vi "Sequencer.min.vi"() -> ()   [LabVIEW 2014]
uses:
  <vilib>/Analysis/NI_AALPro.lvlib
panel:
  in  "Trigger":bool
  out "Counts":u32[](array[numeric])
  out "PMT4":u32[](array[numeric])
  out "PMT3":u32[](array[numeric])
  out "PMT2":u32[](array[numeric])
  out "PMT1":u32[](array[numeric])
  in  "Threshold":dbl=1.0
  out "CompiledSequence":string="#DopplerCooling\r\n0.9 10100000 00000000 00000000\r\n\r\n#Pump\r\n0.3 01000000 00000000 00000000\r\n\r\n#Pulsed\r\n0.2 00100000 00000000 00000000\r\n0.4 00000100 00000000 00000000\r\n0.2 00000000 10000000 00000000\r\n0.2 01000000 00000000 01000000\n"
  out "ChapterNames":string[](array[string])
  out "ChapterPositions":u32[](array[numeric])
  in  "Scan":enum32{"Time"}(tab)
  out "Now (us)":dbl=1.0 format="%.2f"
  in  "Step (us)":dbl=1.0 format="%.2f"
  in  "End (us)":dbl=1.0 format="%.2f"
  in  "Start (us)":dbl=1.0 format="%.2f"
  in  "Time Scan":bool
  in  "Chapter":u16(ring) items=["Zero", "Cooling[0]", "Cooling[1]", "Cooling[2]", "Zero"]
  in  "Once":bool=TRUE
  in  "Sequencer Port":refnum<visa-resource-name>="COM5"
  in  "Send":bool
  out "Durations Backup":dbl[](array[numeric])
  out "Durations":dbl[](array[numeric])
  in  "Period (ns)":dbl=5.0
  out "States":string[](array[string])
  in  "Sequencer":bool
  in  "Edit":enum32{"Sequence"}(tab)
  in  "Sequence":string
  in  "Save":bool
  in  "Chapter (us)":string
  in  "Sequence File":path=path "E:/Data/Sequence/Cooling.seq"
  in  "Repeats":u32=100
  in  "Compile":bool
  in  "Data":bool
  out "Clock":string
  in  "Detect":enum32{"PMT", "TTL"}(tab)
  in  "4":bool
  in  "3":bool
  in  "2":bool
  in  "1":bool=TRUE
  in  "Save":bool
  in  "Count or State":i16(ring) items=["Count", "State"]
  in  "Fit":bool
  out "Peak":u32
  out "?":cluster{dbl[], "Axis":dbl[]}(graph)
  out "?":cluster{"Axis":dbl[], "Histogram":i32[]}(graph)
  in  "Data Chapter":i16(ring) items=["All", "Cooling[2]"]
  out "Average Counts or States":dbl(graph)
  out "Average of Scans":dbl[](graph)
  out "data file":string
  out "History Data":dbl[](array[numeric])
  in  "Sweep":bool
  in  "Clear":bool
  out "Digital Waveform Graph":digitaldata(graph)
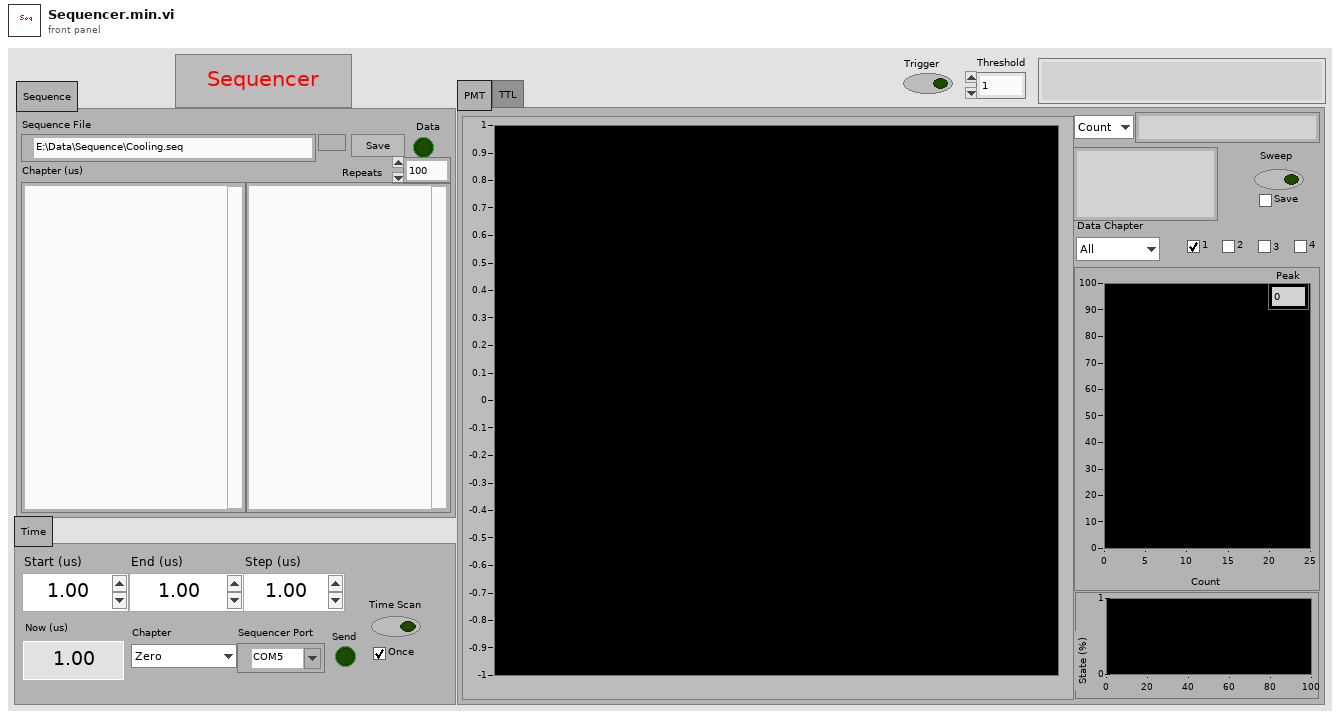
[diagram p1: front panel]
types:
  T1 = cluster{"lower":dbl, "upper":dbl, "inclusion":enum32{"lower", "upper", "both", "neither"}}[]
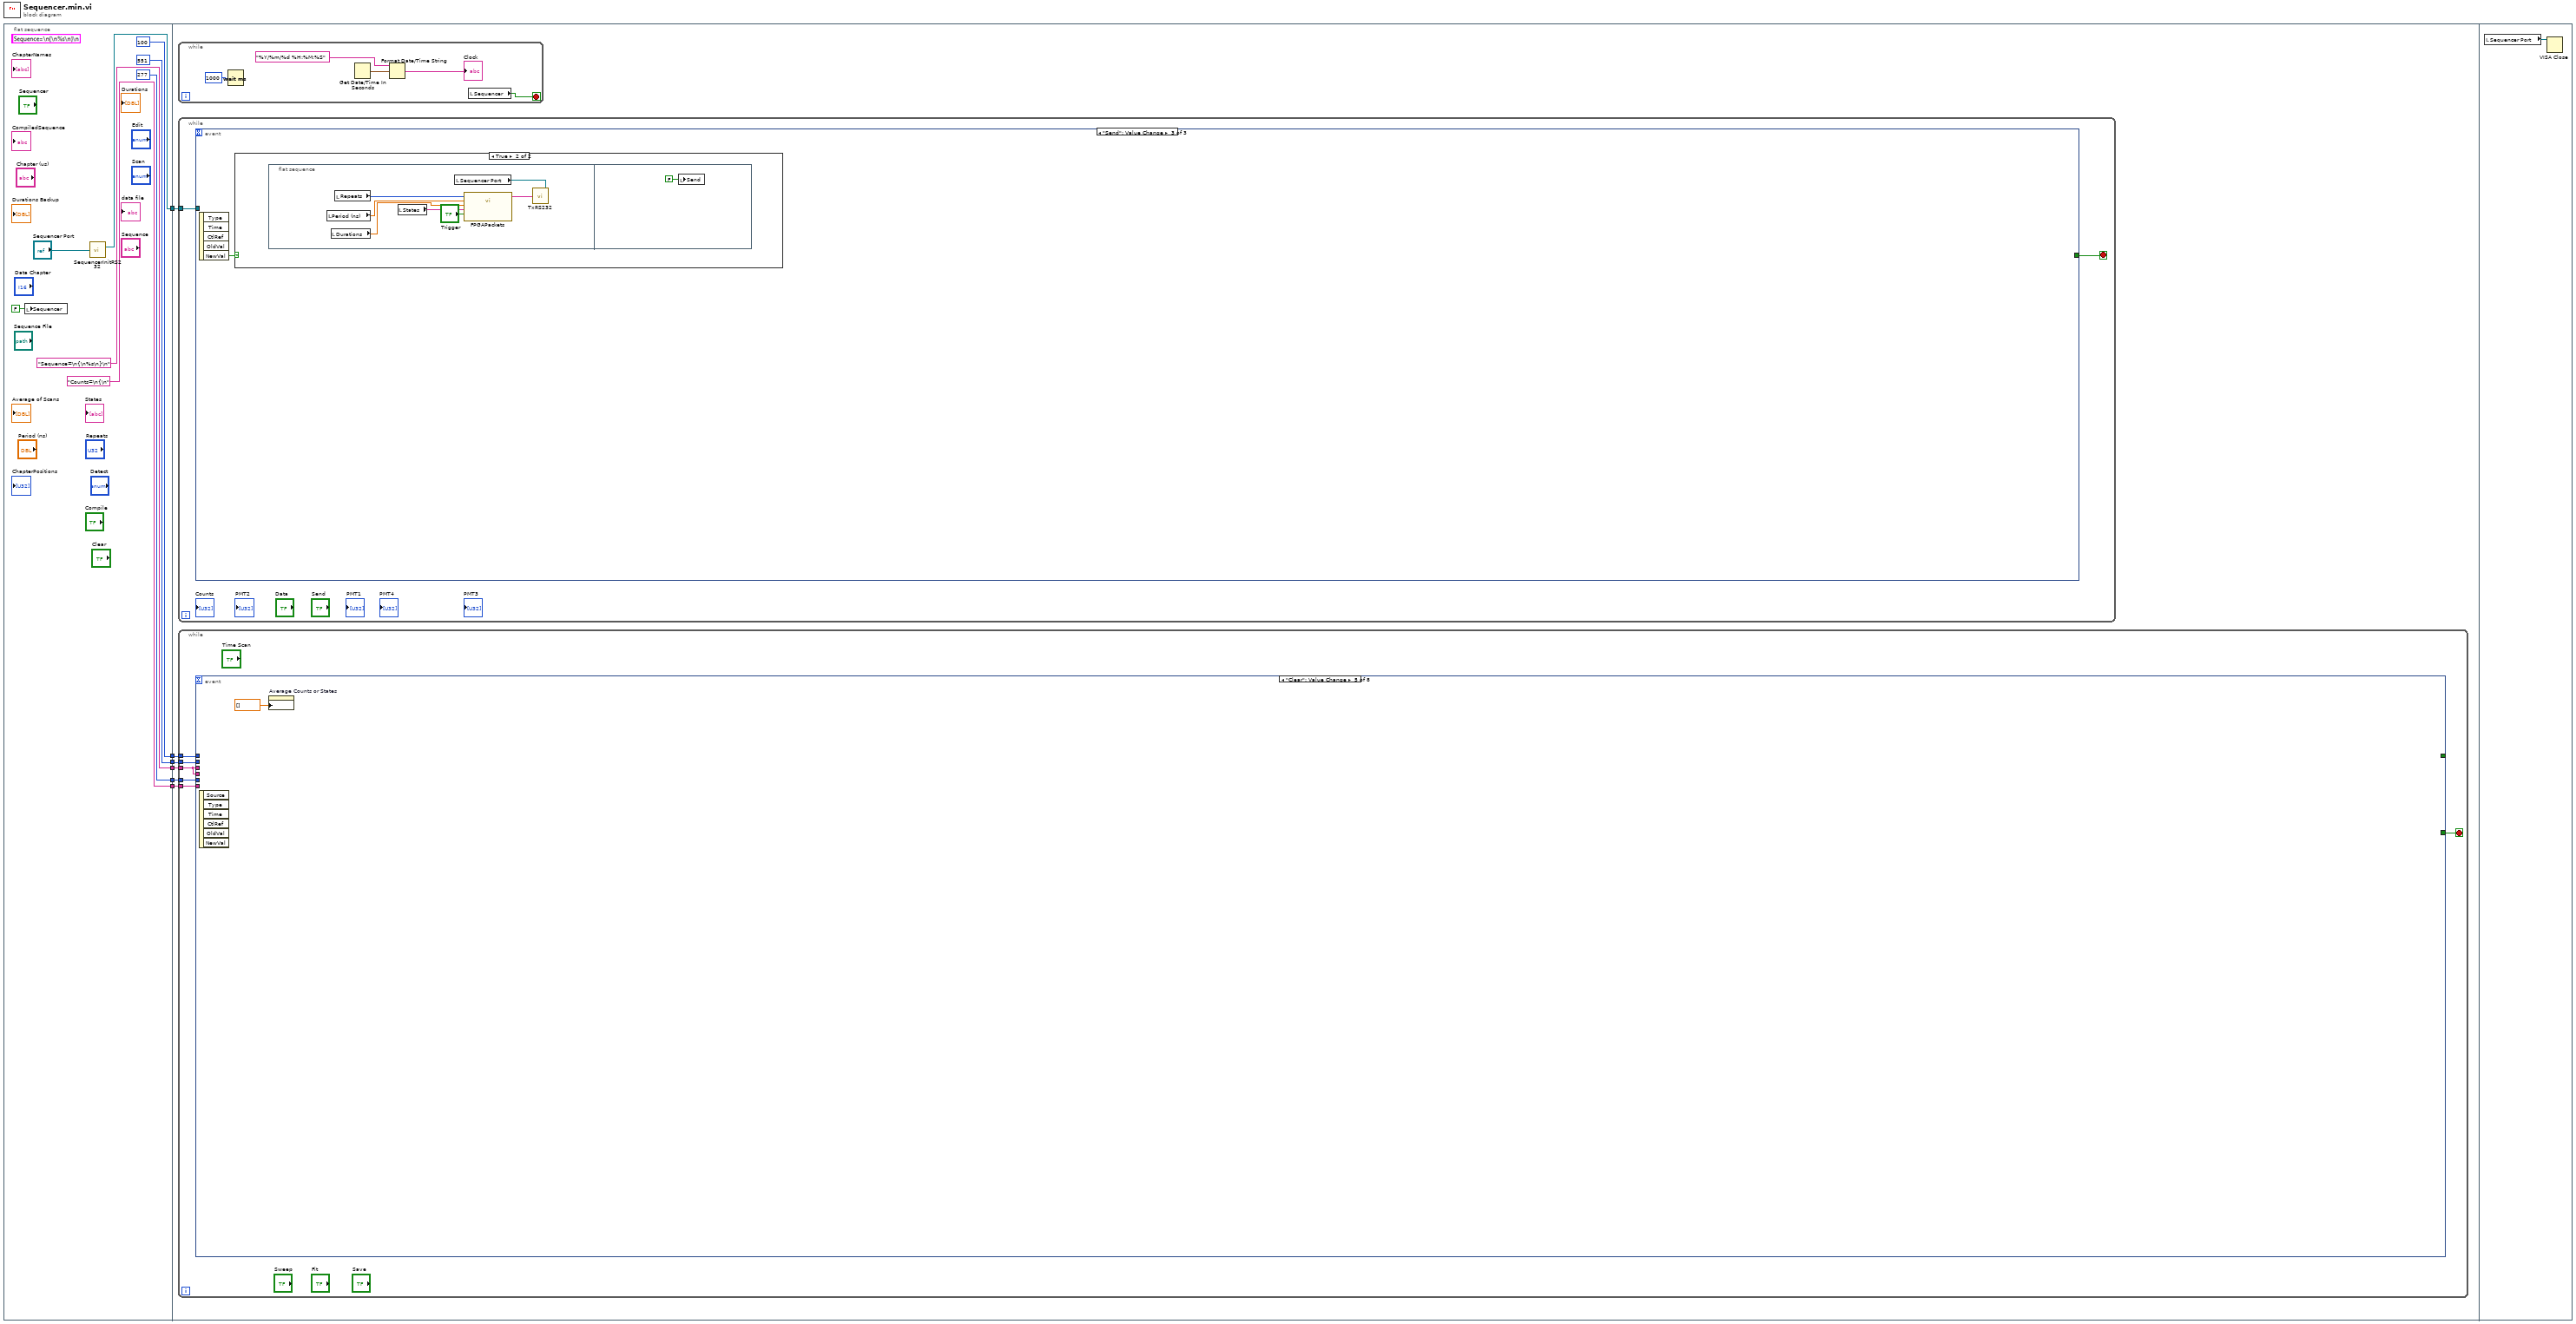
[diagram p0: block diagram]
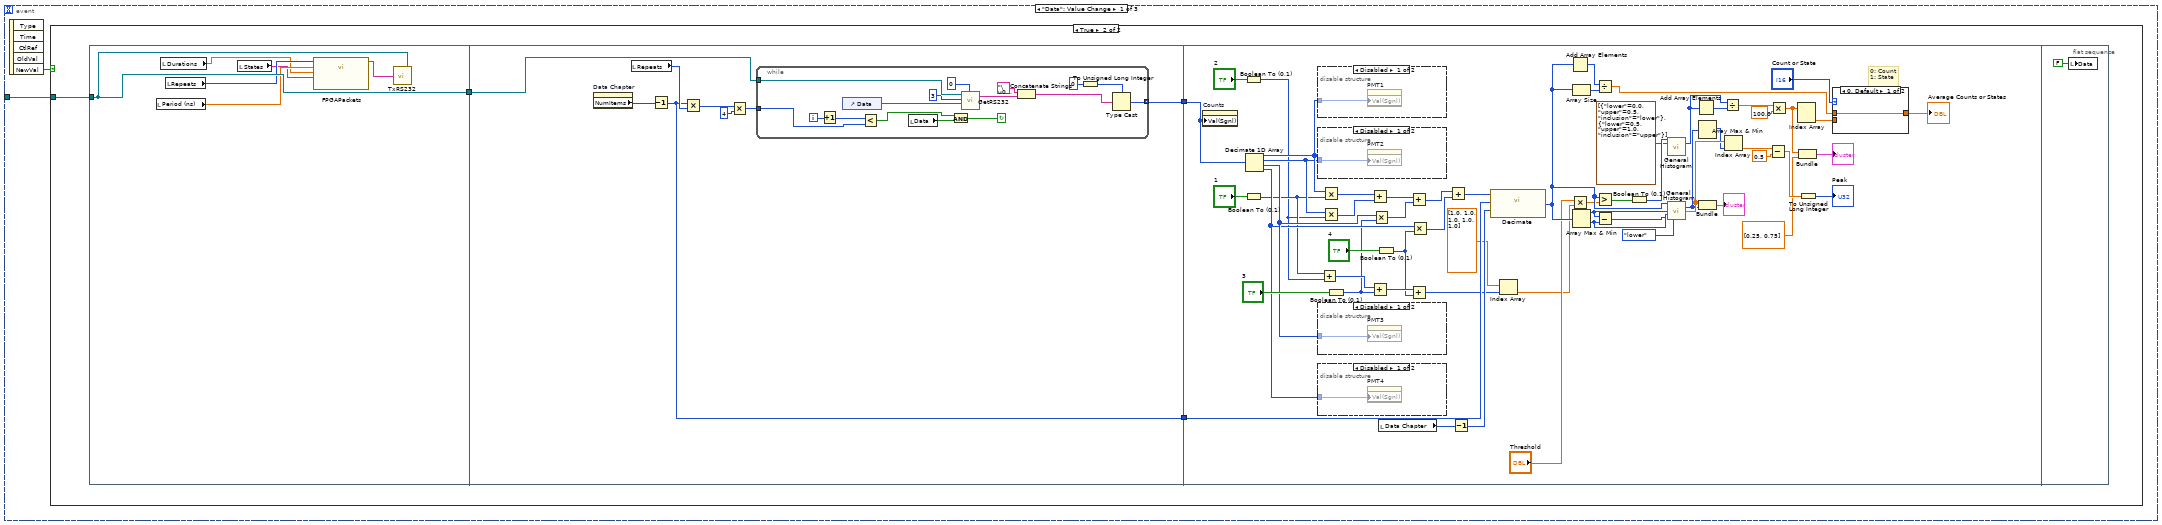
[diagram p2: hidden frame]
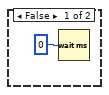
[diagram p3: hidden frame]
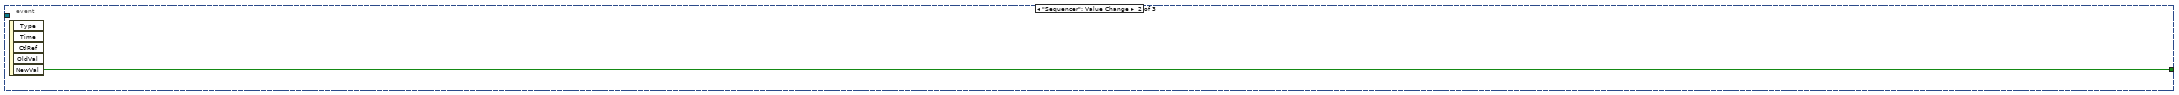
[diagram p9: hidden frame]
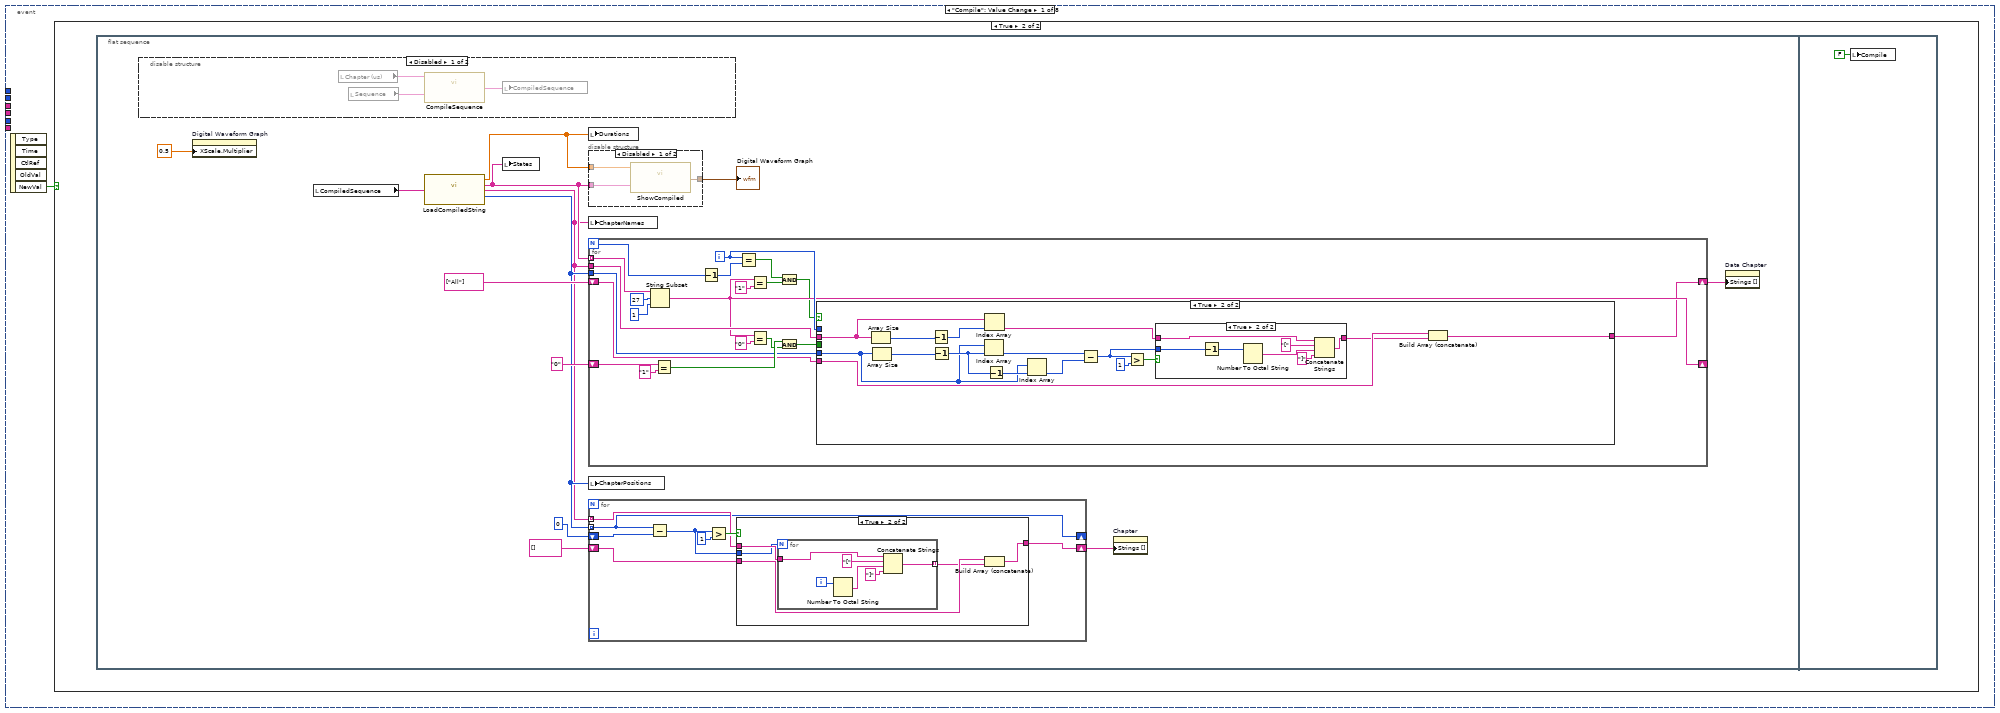
[diagram p11: hidden frame]
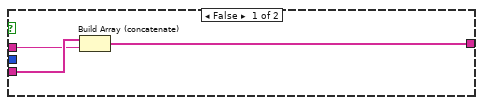
[diagram p15: hidden frame]
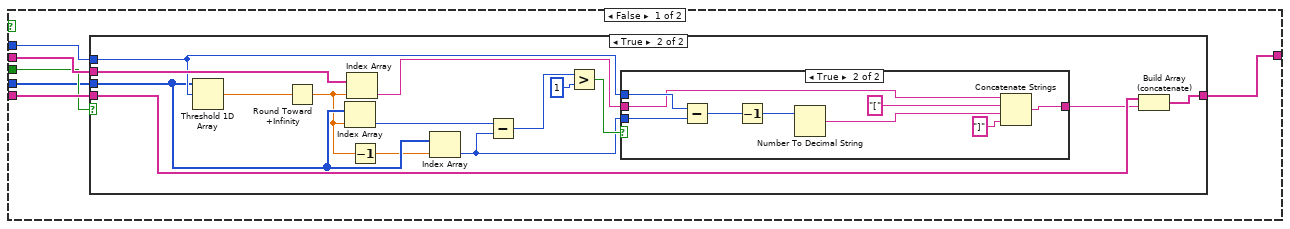
[diagram p16: hidden frame]
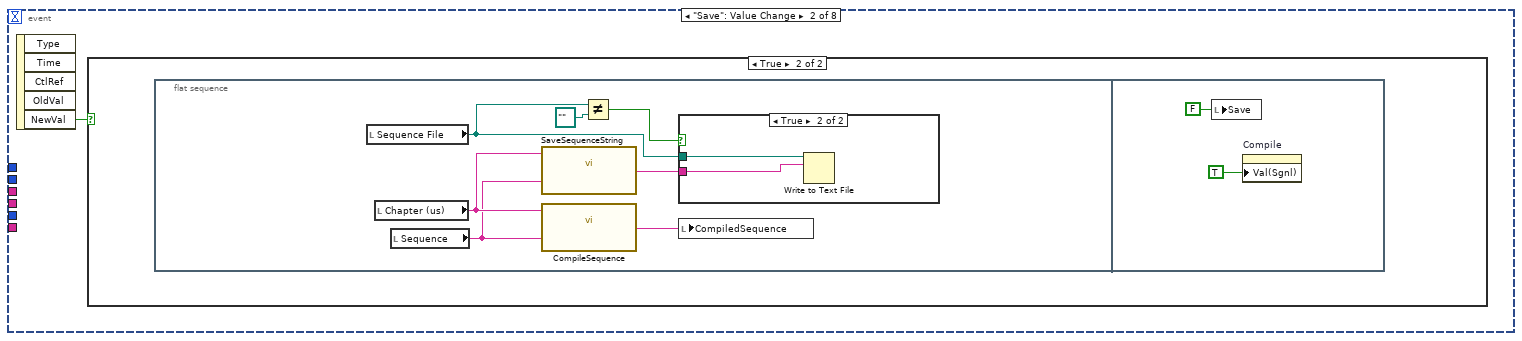
[diagram p20: hidden frame]
diagram:
  n1 = flat-sequence {
    tunnel: [w7] -> w6
    tunnel: [u32 277 ("XControl:Container Bounds:Height")] -> w5
    tunnel: [u32 551 ("Plot Area:Size:Height")] -> w4
    tunnel: [100 ("y")] -> w3
    tunnel: ["Sequence=\n{\n%s\n}\n" ("format string")] -> w2
    tunnel: ["Counts=\n{\n" ("text")] -> w1
    tunnel: w6 -> [w20]
    tunnel: w5 -> [w19]
    tunnel: w4 -> [w18]
    tunnel: w3 -> [w17]
    tunnel: w2 -> [w16]
    tunnel: w1 -> [w15]
    frame #0 {
      n2 = local write "Sequencer"(FALSE ("Sequencer")) -> ()
      n3 = call "SequencerInitRS232.vi"("VISA resource name"="Sequencer Port") -> ("reference out"=w7:refnum<visa-resource-name>)  [unwired: 1 out]
    }
    frame #1 {
      n4 = while {
        stop <- w21 stop-if-true
        n5 = Wait (ms)(milliseconds to wait=u32 1000) -> ()  [unwired: 1 out]
        n6 = Get Date/Time In Seconds() -> (seconds since 1Jan1904=w25:timestamp)
        n7 = Format Date/Time String(time format string (%c)="%Y/%m/%d %H:%M:%S", seconds (now)=w25) -> (date/time string=→"Clock":string)  [unwired: 1 in]
        n8 = local read "Sequencer"() -> (w21:bool)
      }
      n9 = while {
        tunnel: w20 -> [w27]
        stop <- w26 stop-if-true
        n10 = event shown="[2] \"Send\": Value Change" {
          selector: _ -> [_ _ _]
          dyn-events: _ -> [_ _ _]
          timeout: _ -> [_ _ _]
          tunnel: w27 -> [w29 _ _]
          tunnel: [_ w131 _] -> w26
          event "Data": Value Change {
            n11 = event-data() -> ("NewVal"=w28:bool)  [unwired: 1 in, 4 out]
            n12 = case shown="True" w28 {
              tunnel: w29 -> [_ w34]
              frame False {
                n13 = Wait (ms)(milliseconds to wait=u32 0) -> ()  [unwired: 1 out]
              }
              frame True {
                n14 = flat-sequence {
                  tunnel: w34 -> [w39]
                  tunnel: [w39] -> w31
                  tunnel: [w46] -> w33
                  tunnel: [w44] -> w32
                  tunnel: w31 -> [w48]
                  tunnel: w33 -> [w91]
                  tunnel: w32 -> [w97]
                  frame #0 {
                    n15 = local read "Period (ns)"() -> (w37:dbl)
                    n16 = local read "Durations"() -> (w36:dbl[])
                    n17 = local read "Repeats"() -> (w38:u32)
                    n18 = local read "States"() -> (w35:string[])
                    n19 = call "FPGAPackets.vi"("Repeats"=w38, "Period (ns)"=w37, "Durations"=w36, "States"=w35) -> ("Packets"=w40:string)  [unwired: 1 in, 1 out]
                    n20 = call "TxRS232.vi"("VISA resource name"=w39, "Data"=w40) -> ()
                  }
                  frame #1 {
                    n21 = property on="Data Chapter" class="Ring (strict)"() -> ("NumItems"=w47:u32)  [unwired: 2 in, 2 out]
                    n22 = local read "Repeats"() -> (w45:u32)
                    n23 = Decrement(x=w47) -> (x-1=w44:u32)
                    n24 = Multiply(x=w44, y=w45) -> (x*y=w43:u32)
                    n25 = Multiply(x=w43, y=u32 4) -> (x*y=w42:u32)
                    n26 = while {
                      tunnel: w48 -> [w56]
                      tunnel: [w57] -> w46 mode=indexing
                      tunnel: w42 -> [w52]
                      i -> [w51]
                      stop <- w60 continue-if-true
                      n27 = Increment(x=w51) -> (x+1=w50:i32)
                      n28 = control-ref of="Data"() -> (w53:refnum<vi>)
                      n29 = Less?(x=w50, y=w52) -> (x < y?=w59:bool)
                      n30 = local read "Data"() -> (w61:bool)
                      n31 = And(x=w59, y=w61) -> (x .and. y?=w60:bool)
                      n32 = call "GetRS232.vi"("VISA resource name"=w56, "Bytes To Read"=3, "Control"=w53, "Limit"=0) -> ("Data"=w54:string)  [unwired: 1 in, 1 out]
                      n33 = Concatenate Strings("\u0000" ("string"), w54) -> (w58:string)
                      n34 = To Unsigned Long Integer(number=u32 0) -> (unsigned 32bit integer=w64:u32)
                      n35 = Type Cast(type=w64, x=w58) -> (*(type *) &x=w57:u32)
                    }
                  }
                  frame #2 {
                    # "0: Count\n1: State"
                    n36 = property on="Counts" class="Arr (strict)"("Val(Sgnl)"=w91) -> ()  [unwired: 2 in, 2 out]
                    n37 = Boolean To (0,1)(Boolean="2") -> (0, 1=w74:i16)
                    n38 = Boolean To (0,1)(Boolean="1") -> (0, 1=w75:i16)
                    n39 = Decimate 1D Array(w91) -> (w90:u32[], w87:u32[], w83:u32[], w80:u32[])
                    n40 = disable-structure shown="Disabled" {
                      disable-tunnel: w90 -> [w127 _]
                      frame Disabled {
                        n41 = property on="PMT1" class="Arr (strict)"("Val(Sgnl)"=w127) -> ()  [unwired: 2 in, 2 out]
                      }
                      frame Enabled {
                      }
                    }
                    n42 = disable-structure shown="Disabled" {
                      disable-tunnel: w87 -> [w126 _]
                      frame Disabled {
                        n43 = property on="PMT2" class="Arr (strict)"("Val(Sgnl)"=w126) -> ()  [unwired: 2 in, 2 out]
                      }
                      frame Enabled {
                      }
                    }
                    n44 = disable-structure shown="Disabled" {
                      disable-tunnel: w83 -> [w125 _]
                      frame Disabled {
                        n45 = property on="PMT3" class="Arr (strict)"("Val(Sgnl)"=w125) -> ()  [unwired: 2 in, 2 out]
                      }
                      frame Enabled {
                      }
                    }
                    n46 = disable-structure shown="Disabled" {
                      disable-tunnel: w80 -> [w124 _]
                      frame Disabled {
                        n47 = property on="PMT4" class="Arr (strict)"("Val(Sgnl)"=w124) -> ()  [unwired: 2 in, 2 out]
                      }
                      frame Enabled {
                      }
                    }
                    n48 = Add(x=w75, y=w74) -> (x+y=w73:i16)
                    n49 = Multiply(x=w90, y=w75) -> (x*y=w76:u32[])
                    n50 = Multiply(x=w87, y=w74) -> (x*y=w86:u32[])
                    n51 = Boolean To (0,1)(Boolean="3") -> (0, 1=w72:i16)
                    n52 = Add(x=w76, y=w86) -> (x+y=w81:u32[])
                    n53 = Add(x=w73, y=w72) -> (x+y=w71:i16)
                    n54 = Multiply(x=w83, y=w72) -> (x*y=w82:u32[])
                    n55 = Boolean To (0,1)(Boolean="4") -> (0, 1=w70:i16)
                    n56 = local read "Data Chapter"() -> (w95:i16)
                    n57 = Add(x=w81, y=w82) -> (x+y=w78:u32[])
                    n58 = Add(x=w71, y=w70) -> (x+y=w65:i16)
                    n59 = Multiply(x=w80, y=w70) -> (x*y=w79:u32[])
                    n60 = Add(x=w78, y=w79) -> (x+y=w77:u32[])
                    n61 = Decrement(x=w95) -> (x-1=w94:i16)
                    n62 = call "Decimate.vi"("i"=w94, "n"=w97, "Input Array"=w77) -> ("Decimated Array"=w119:u32[])
                    n63 = Index Array(array=dbl[] [1.0, 1.0, 1.0, 1.0, 1.0], index=w65) -> (element=w67:dbl)
                    n64 = Add Array Elements(numeric array=w119) -> (sum=w118:u32)
                    n65 = Multiply(x="Threshold", y=w67) -> (x*y=w66:dbl)
                    n66 = Array Size(array=w119) -> (size(s)=w117:i32)
                    n67 = Array Max & Min(array=w119) -> (max value=w98:u32, min value=w108:u32)  [unwired: 2 out]
                    n68 = Divide(x=w118, y=w117) -> (x/y=w121:dbl)
                    n69 = Greater?(x=w119, y=w66) -> (0:w104:bool[])
                    n70 = Subtract(x=w98, y=w108) -> (x-y=w107:u32)
                    n71 = Boolean To (0,1)(Boolean=w104) -> (0, 1=w103:i16[])
                    n72 = call <vilib>:"General Histogram.vi"("X"=w103, "Bins"=T1 [{"lower"=0.0, "upper"=0.5, "inclusion"=enum."lower"}, {"lower"=0.5, "upper"=1.0, "inclusion"=enum."upper"}]) -> ("Histogram"=w101:i32[])  [unwired: 9 in, 4 out]
                    n73 = call <vilib>:"General Histogram.vi"("X"=w119, "max"=w98, "min"=w108, "# bins"=w107, "inclusion"=enum32{"lower", "upper"}."lower") -> ("Histogram"=w109:i32[], "Axis"=w111:dbl[])  [unwired: 6 in, 3 out]
                    n74 = Add Array Elements(numeric array=w101) -> (sum=w102:i32)
                    n75 = Array Max & Min(array=w109) -> (max index (indices)=w110:i32)  [unwired: 3 out]
                    n76 = Bundle("Axis"=w111, "Histogram"=w109) -> (→"?":cluster{"Axis":dbl[], "Histogram":i32[]})  [unwired: 1 in]
                    n77 = Divide(x=w101, y=w102) -> (x/y=w99:dbl[])
                    n78 = Index Array(array=w111, index=w110) -> (element=w115:dbl)
                    n79 = Subtract(x=w115, y=0.5) -> (x-y=w114:dbl)
                    n80 = Multiply(x=w99, y=100.0) -> (x*y=w120:dbl[])
                    n81 = Index Array(array=w120) -> (element #2=w122:dbl)  [unwired: 2 in, 1 out]
                    n82 = Bundle(w120, "Axis"=dbl[] [0.25, 0.75]) -> (→"?":cluster{dbl[], "Axis":dbl[]})  [unwired: 1 in]
                    n83 = To Unsigned Long Integer(number=w114) -> (unsigned 32bit integer=→"Peak":u32)
                    n84 = case shown="0, Default" "Count or State" {
                      tunnel: w121 -> [w128 _]
                      tunnel: [w128 w129] -> w123
                      tunnel: w122 -> [_ w129]
                      frame 0, Default {
                      }
                      frame 1 {
                      }
                    }
                    "Average Counts or States" <- w123
                  }
                  frame #3 {
                    n85 = local write "Data"(FALSE ("Acquisition")) -> ()
                  }
                }
              }
            }
          }
          event "Sequencer": Value Change {
            n86 = event-data() -> ("NewVal"=w131:bool)  [unwired: 1 in, 4 out]
          }
          event "Send": Value Change {
            n87 = event-data() -> ("NewVal"=w132:bool)  [unwired: 1 in, 4 out]
            n88 = case shown="True" w132 {
              frame False {
              }
              frame True {
                n89 = flat-sequence {
                  frame #0 {
                    n90 = local read "Period (ns)"() -> (w137:dbl)
                    n91 = local read "Durations"() -> (w135:dbl[])
                    n92 = local read "Repeats"() -> (w136:u32)
                    n93 = local read "States"() -> (w138:string[])
                    n94 = local read "Sequencer Port"() -> (w139:refnum<visa-resource-name>)
                    n95 = call "FPGAPackets.vi"("Repeats"=w136, "Period (ns)"=w137, "Durations"=w135, "States"=w138, "Trigger"="Trigger") -> ("Packets"=w134:string)  [unwired: 1 out]
                    n96 = call "TxRS232.vi"("VISA resource name"=w139, "Data"=w134) -> ()
                  }
                  frame #1 {
                    n97 = local write "Send"(FALSE ("Send")) -> ()
                  }
                }
              }
            }
          }
        }
      }
      n98 = while {
        tunnel: w19 -> [w145]
        tunnel: w18 -> [w144]
        tunnel: w17 -> [w143]
        tunnel: w16 -> [w141]
        tunnel: w15 -> [w142]
        stop <- w146 stop-if-true
        n99 = event shown="[4] \"Clear\": Value Change" {
          selector: _ -> [_ _ _ _ _ _ _ _]
          dyn-events: _ -> [_ _ _ _ _ _ _ _]
          timeout: _ -> [_ _ _ _ _ _ _ _]
          tunnel: [_ _ _ _ _ _ _ w497] -> _
          tunnel: [_ _ _ _ _ _ _ w497] -> w146
          tunnel: w145 -> [_ _ w280 _ _ _ _ _]
          tunnel: w144 -> [_ _ _ _ _ _ w434 _]
          tunnel: w143 -> [_ _ _ _ _ _ w433 _]
          tunnel: w141 -> [_ _ _ _ _ _ w432 _]
          tunnel: w142 -> [_ _ _ _ _ _ w431 _]
          tunnel: w141 -> [_ _ w279 _ _ _ _ _]
          event "Compile": Value Change {
            n100 = event-data() -> ("NewVal"=w147:bool)  [unwired: 1 in, 4 out]
            n101 = case shown="True" w147 {
              frame False {
              }
              frame True {
                n102 = flat-sequence {
                  frame #0 {
                    n103 = disable-structure shown="Disabled" {
                      frame Disabled {
                        n104 = local read "Chapter (us)"() -> (w166:string)
                        n105 = local read "Sequence"() -> (w165:string)
                        n106 = call "CompileSequence.vi"("Sequence"=w165, "Chapter"=w166) -> ("Compiled Sequence"=w164:string)
                        n107 = local write "CompiledSequence"(w164) -> ()
                      }
                      frame Enabled {
                      }
                    }
                    n108 = property on="Digital Waveform Graph" class="DigitalGraph (strict)"("XScale.Multiplier"=0.5 ("X Scale.Offset and Multiplier:Multiplier")) -> ()  [unwired: 2 in, 2 out]
                    n109 = local read "CompiledSequence"() -> (w148:string)
                    n110 = call "LoadCompiledString.vi"("Compiled String"=w148) -> ("Durations"=w159:dbl[], "States"=w158:string[], "ChapterNames"=w149:string[], "ChapterPositions"=w150:u32[])
                    n111 = local write "States"(w158) -> ()
                    n112 = local write "Durations"(w159) -> ()
                    n113 = disable-structure shown="Disabled" {
                      disable-tunnel: [w163 _] -> w160
                      disable-tunnel: w159 -> [w162 _]
                      disable-tunnel: w158 -> [w161 _]
                      frame Disabled {
                        n114 = call "ShowCompiled.vi"("States"=w161, "Durations"=w162) -> ("Digital Waveform Graph"=w163:digitaldata)
                      }
                      frame Enabled {
                      }
                    }
                    "Digital Waveform Graph" <- w160
                    n115 = local write "ChapterNames"(w149) -> ()
                    n116 = for {
                      N -> [w200]
                      tunnel: w158 -> [w209] mode=indexing
                      shift-right: [w197] -> _
                      shift-left: "0" -> [w207]
                      tunnel: w149 -> [w203]
                      shift-right: [w192] -> w153
                      shift-left: string[] ["All"] -> [w191]
                      tunnel: w150 -> [w190]
                      i -> [w201]
                      n117 = String Subset(string=w209, offset (0)=27, length (rest)=1 ("length (rest)")) -> (substring=w197:string)
                      n118 = Equal?(x=w207, y="1") -> (x = y?=w205:bool)
                      n119 = Decrement(x=w200) -> (x-1=w199:i32)
                      n120 = Equal?(x=w201, y=w199) -> (x = y?=w196:bool)
                      n121 = Equal?(x=w197, y="1") -> (x = y?=w195:bool)
                      n122 = Equal?(x=w197, y="0") -> (x = y?=w202:bool)
                      n123 = And(x=w196, y=w195) -> (x .and. y?=w194:bool)
                      n124 = And(x=w205, y=w202) -> (x .and. y?=w193:bool)
                      n125 = case shown="True" w194 {
                        tunnel: w203 -> [w215 w255]
                        tunnel: w191 -> [w214 w257]
                        tunnel: w201 -> [w213 _]
                        tunnel: w193 -> [w212 _]
                        tunnel: [w211 w256] -> w192
                        tunnel: w190 -> [w210 w249]
                        frame False {
                          n126 = case shown="True" w212 {
                            tunnel: w213 -> [_ w227]
                            tunnel: w215 -> [_ w228]
                            tunnel: w214 -> [w216 w230]
                            tunnel: [w216 w231] -> w211
                            tunnel: w210 -> [_ w224]
                            frame False {
                            }
                            frame True {
                              n127 = Threshold 1D Array(2:w227, 3:w224) -> (0:w229:dbl)  [unwired: 1 in]
                              n128 = Round Toward +Infinity(x=w229) -> (ceil(x): smallest int >= x=w222:dbl)
                              n129 = Index Array(array=w224, index=w222) -> (element=w221:u32)
                              n130 = Index Array(array=w228, index=w222) -> (element=w225:string)
                              n131 = Decrement(x=w222) -> (x-1=w223:dbl)
                              n132 = Index Array(array=w224, index=w223) -> (element=w217:u32)
                              n133 = Subtract(x=w221, y=w217) -> (x-y=w220:u32)
                              n134 = Greater?(x=w220, y=u32 1) -> (0:w218:bool)
                              n135 = case shown="True" w218 {
                                tunnel: w227 -> [_ w241]
                                tunnel: [w232 w235] -> w226
                                tunnel: w225 -> [w232 w234]
                                tunnel: w217 -> [_ w233]
                                frame False {
                                }
                                frame True {
                                n136 = Subtract(x=w241, y=w233) -> (x-y=w240:u32)
                                n137 = Decrement(x=w240) -> (x-1=w239:u32)
                                n138 = Number To Decimal String(number=w239) -> (decimal integer string=w236:string)  [unwired: 1 in]
                                n139 = Concatenate Strings(w234, "[" ("element"), w236, "]" ("element")) -> (w235:string)
                                }
                              }
                              n140 = Build Array (concatenate)(w230, w226) -> (w231:string[])
                            }
                          }
                        }
                        frame True {
                          n141 = Array Size(array=w255) -> (size(s)=w254:i32)
                          n142 = Array Size(array=w249) -> (size(s)=w252:i32)
                          n143 = Decrement(x=w254) -> (x-1=w253:i32)
                          n144 = Decrement(x=w252) -> (x-1=w251:i32)
                          n145 = Index Array(array=w249, index=w251) -> (element=w248:u32)
                          n146 = Index Array(array=w255, index=w253) -> (element=w244:string)
                          n147 = Decrement(x=w251) -> (x-1=w250:i32)
                          n148 = Index Array(array=w249, index=w250) -> (element=w247:u32)
                          n149 = Subtract(x=w248, y=w247) -> (x-y=w242:u32)
                          n150 = Greater?(x=w242, y=u32 1) -> (0:w245:bool)
                          n151 = case shown="True" w245 {
                            tunnel: w244 -> [w258 w265]
                            tunnel: [w258 w259] -> w243
                            tunnel: w242 -> [_ w262]
                            frame False {
                            }
                            frame True {
                              n152 = Decrement(x=w262) -> (x-1=w261:u32)
                              n153 = Number To Octal String(2:w261) -> (0:w260:string)  [unwired: 1 in]
                              n154 = Concatenate Strings(w265, "[" ("string"), w260, "]" ("string")) -> (w259:string)
                            }
                          }
                          n155 = Build Array (concatenate)(w257, w243) -> (w256:string[])
                        }
                      }
                    }
                    n156 = local write "ChapterPositions"(w150) -> ()
                    n157 = for {
                      tunnel: w150 -> [w167] mode=indexing
                      tunnel: w149 -> [w168] mode=indexing
                      shift-right: [w167] -> _
                      shift-left: u32 0 ("initial scan location") -> [w174]
                      shift-right: [w169] -> w155
                      shift-left: string[] [] -> [w170]
                      n158 = Subtract(x=w167, y=w174) -> (x-y=w171:u32)
                      n159 = Greater?(x=w171, y=u32 1) -> (0:w173:bool)
                      n160 = case shown="True" w173 {
                        tunnel: w168 -> [w176 w182]
                        tunnel: w171 -> [_ w181]
                        tunnel: w170 -> [w177 w180]
                        tunnel: [w175 w178] -> w169
                        frame False {
                          n161 = Build Array (concatenate)(w177, w176) -> (w175:string[])
                        }
                        frame True {
                          n162 = for {
                            N: w181 -> [_]
                            tunnel: w182 -> [w187]
                            tunnel: [w186] -> w179 mode=indexing
                            i -> [w188]
                            n163 = Number To Octal String(2:w188) -> (0:w185:string)  [unwired: 1 in]
                            n164 = Concatenate Strings(w187, "[" ("string"), w185, "]" ("string")) -> (w186:string)
                          }
                          n165 = Build Array (concatenate)(w180, w179) -> (w178:string[])
                        }
                      }
                    }
                    n166 = property on="Chapter" class="Ring (strict)"("Strings []"=w155) -> ()  [unwired: 2 in, 2 out]
                    n167 = property on="Data Chapter" class="Ring (strict)"("Strings []"=w153) -> ()  [unwired: 2 in, 2 out]
                  }
                  frame #1 {
                    n168 = local write "Compile"(FALSE ("Compile")) -> ()
                  }
                }
              }
            }
          }
          event "Save": Value Change {
            n169 = event-data() -> ("NewVal"=w267:bool)  [unwired: 1 in, 4 out]
            n170 = case shown="True" w267 {
              frame False {
              }
              frame True {
                n171 = flat-sequence {
                  frame #0 {
                    n172 = local read "Sequence File"() -> (w272:path)
                    n173 = local read "Chapter (us)"() -> (w270:string)
                    n174 = local read "Sequence"() -> (w269:string)
                    n175 = call "SaveSequenceString.vi"("Sequence"=w269, "Chapter"=w270) -> ("Sequence String"=w271:string)
                    n176 = call "CompileSequence.vi"("Sequence"=w269, "Chapter"=w270) -> ("Compiled Sequence"=w268:string)
                    n177 = Not Equal?(x=w272, y=path "") -> (x != y?=w274:bool)
                    n178 = case shown="True" w274 {
                      tunnel: w272 -> [_ w276]
                      tunnel: w271 -> [_ w275]
                      frame False {
                      }
                      frame True {
                        n179 = Write to Text File(file (use dialog)=w276, text=w275) -> ()  [unwired: 2 in, 3 out]
                      }
                    }
                    n180 = local write "CompiledSequence"(w268) -> ()
                  }
                  frame #1 {
                    n181 = local write "Save"(FALSE ("Compile")) -> ()
                    n182 = property on="Compile" class="Bool (strict)"("Val(Sgnl)"=TRUE ("Value (Signaling)")) -> ()  [unwired: 2 in, 2 out]
                  }
                }
              }
            }
          }
          event "Time Scan": Value Change {
            n183 = event-data() -> ("NewVal"=w281:bool)  [unwired: 1 in, 4 out]
            n184 = case shown="True" w281 {
              tunnel: w280 -> [_ w293]
              tunnel: w279 -> [_ w286]
              frame False {
                n185 = local read "Durations Backup"() -> (w282:dbl[])
                n186 = local write "Durations"(w282) -> ()
              }
              frame True {
                (unwired) "," ("delimiter (Tab)")
                w306 = " us" ("string")
                w303 = "\r\n"
                n187 = property on="Average Counts or States" class="WFChart (strict)"("Height"=w293, "History Data"=dbl[] []) -> (error out=w292:errorcluster)  [unwired: 2 in, 1 out]
                n188 = local read "Chapter (us)"() -> (w313:string)
                n189 = local read "Sequence"() -> (w314:string)
                n190 = property on="Average of Scans" class="WFGraph (strict)"("XScale.Multiplier"="Step (us)", "XScale.Offset"="Start (us)", "XScale.Maximum"="End (us)") -> ()  [unwired: 2 in, 2 out]
                n191 = Subtract(x="End (us)", y="Start (us)") -> (x-y=w321:dbl)
                n192 = Number To Decimal String(number="Chapter") -> (decimal integer string=w317:string)  [unwired: 1 in]
                n193 = Number To Fractional String(number="Start (us)") -> (F-format string=w311:string)  [unwired: 3 in]
                n194 = Number To Fractional String(number="End (us)") -> (F-format string=w309:string)  [unwired: 3 in]
                n195 = Number To Fractional String(number="Step (us)") -> (F-format string=w307:string)  [unwired: 3 in]
                n196 = call "NewData.vi"("Prefix"="TimeScan-" ("string")) -> ("data file name"=w290:string, "data file refnum"=w284:refnum<file>)  [unwired: 2 in]
                n197 = call "SaveSequenceString.vi"("Sequence"=w314, "Chapter"=w313) -> ("Sequence String"=w285:string)
                n198 = Divide(x=w321, y="Step (us)") -> (x/y=w320:dbl)
                n199 = local write "data file"(w290) -> ()
                n200 = Concatenate Strings("Chapter=" ("string"), w317, w303, "Start=" ("string"), w311, w306, w303, "End=" ("string"), w309, w306, w303, "Step=" ("string"), w307, w306, w303, "Counts=" ("string"), w303, "{" ("string"), w303) -> (w315:string)
                n201 = Format Into String(format string=w286, initial string=w284, w285) -> (resulting string=w283:refnum<file>)  [unwired: 1 in, 1 out]
                n202 = Increment(x=w320) -> (x+1=w319:dbl)
                n203 = property on="Average Counts or States" class="WFChart (strict)"(error in=w292, "XScale.Multiplier"="Step (us)", "XScale.Offset"="Start (us)", "XScale.Maximum"="End (us)") -> ()  [unwired: 1 in, 2 out]
                n204 = local read "Durations"() -> (w296:dbl[])
                n205 = Write to Text File(file (use dialog)=w283, text=w315) -> (refnum out=w302:refnum<file>)  [unwired: 2 in, 2 out]
                n206 = Initialize Array(0.0 ("element"), w319) -> (w295:dbl[])
                n207 = local write "Durations Backup"(w296) -> ()
                n208 = while {
                  tunnel: "Start (us)" -> [w347]
                  tunnel: "Step (us)" -> [w346]
                  tunnel: "End (us)" -> [w345]
                  shift-right: [w335] -> _
                  shift-left: w295 -> [w344]
                  tunnel: w319 -> [w331]
                  tunnel: "Chapter" -> [w334]
                  shift-right: [w333] -> w300
                  shift-left: w302 -> [w332]
                  tunnel: w296 -> [w330]
                  i -> [w337]
                  stop <- w323 continue-if-true
                  n209 = flat-sequence {
                    tunnel: w344 -> [w358]
                    tunnel: w345 -> [w359]
                    tunnel: w346 -> [w360]
                    tunnel: w347 -> [w361]
                    tunnel: [w361] -> w343
                    tunnel: [w360] -> w342
                    tunnel: [w359] -> w341
                    tunnel: [w358] -> w340
                    tunnel: w343 -> [w372]
                    tunnel: w342 -> [w371]
                    tunnel: w341 -> [_]
                    tunnel: w340 -> [w370]
                    tunnel: w334 -> [w368]
                    tunnel: w332 -> [w367]
                    tunnel: w330 -> [w365]
                    tunnel: w329 -> [w364]
                    tunnel: [w370] -> w327
                    tunnel: [w369] -> w326
                    tunnel: [w366] -> w325
                    tunnel: [w362] -> w324
                    tunnel: [w411] -> w328
                    tunnel: [w412] -> w333
                    tunnel: [w408] -> w323
                    tunnel: [w413] -> w336
                    tunnel: w327 -> [w413]
                    tunnel: w326 -> [w409]
                    tunnel: w325 -> [w412]
                    tunnel: w324 -> [w411]
                    frame #0 {
                      n210 = property on="Average Counts or States" class="WFChart (strict)"("History Data"=dbl[] []) -> ()  [unwired: 2 in, 2 out]
                    }
                    frame #1 {
                      n211 = Decrement(x=w364) -> (x-1=w363:u32)
                      n212 = while {
                        shift-right: [w385] -> _
                        shift-left: w372 -> [w373]
                        tunnel: w371 -> [w383]
                        tunnel: [w382] -> w369
                        tunnel: w368 -> [w379]
                        tunnel: w367 -> [w380]
                        tunnel: [w381] -> w366
                        tunnel: w365 -> [w378]
                        tunnel: w363 -> [w375]
                        tunnel: [w374] -> w362 mode=indexing
                        i -> [w377]
                        stop <- w384 continue-if-true
                        n213 = local read "Time Scan"() -> (w382:bool)
                        n214 = flat-sequence {
                          tunnel: w379 -> [w389]
                          tunnel: w373 -> [w388]
                          tunnel: w378 -> [w386]
                          tunnel: w373 -> [w400]
                          tunnel: w380 -> [w395]
                          tunnel: [w394] -> w381
                          tunnel: [w392] -> w374
                          frame #0 {
                            n215 = Replace Array Subset(array=w386, new element=w388, index=w389) -> (w387:dbl[])
                            n216 = local write "Durations"(w387) -> ()
                          }
                          frame #1 {
                            n217 = property on="Data" class="Bool (strict)"("Val(Sgnl)"=TRUE ("Acquisition")) -> ()  [unwired: 2 in, 2 out]
                          }
                          frame #2 {
                            n218 = while {
                              stop <- w391 continue-if-true
                              n219 = local read "Data"() -> (w391:bool)
                            }
                          }
                          frame #3 {
                            n220 = Number To Fractional String(number=w400) -> (F-format string=w402:string)  [unwired: 3 in]
                            n221 = local read "Counts"() -> (w393:u32[])
                            n222 = Concatenate Strings(w402, " us," ("string")) -> (w399:string)
                            n223 = for {
                              tunnel: w393 -> [w407] mode=indexing
                              shift-right: [w405] -> w396
                              shift-left: w399 -> [w404]
                              n224 = Number To Decimal String(number=w407) -> (decimal integer string=w406:string)  [unwired: 1 in]
                              n225 = call <vilib>:"Space Constant.vi"() -> ("String"=w403:string)
                              n226 = Concatenate Strings(w404, w403, w406) -> (w405:string)
                            }
                            n227 = local read "Average Counts or States"() -> (w392:dbl)
                            n228 = Concatenate Strings(w396, "\r\n") -> (w397:string)
                            n229 = Write to Text File(file (use dialog)=w395, text=w397) -> (refnum out=w394:refnum<file>)  [unwired: 2 in, 2 out]
                          }
                        }
                        n230 = Add(x=w373, y=w383) -> (x+y=w385:dbl)
                        n231 = Less?(x=w377, y=w375) -> (x < y?=w376:bool)
                        n232 = And(x=w382, y=w376) -> (x .and. y?=w384:bool)
                        "Now (us)" <- w373
                      }
                    }
                    frame #2 {
                      n233 = case shown="True" "Once" {
                        tunnel: w409 -> [w414 _]
                        tunnel: [w414 w416] -> w408
                        frame False {
                        }
                        frame True {
                          w416 = FALSE ("Time Scan")
                          n234 = local read "Durations Backup"() -> (w415:dbl[])
                          n235 = local write "Durations"(w415) -> ()
                          n236 = local write "Time Scan"(w416) -> ()
                        }
                      }
                    }
                  }
                  n237 = To Unsigned Long Integer(number=w331) -> (unsigned 32bit integer=w329:u32)
                  n238 = Array Size(array=w328) -> (size(s)=w338:i32)
                  n239 = Equal?(x=w338, y=w329) -> (x = y?=w339:bool)
                  n240 = case shown="True" w339 {
                    tunnel: w337 -> [_ w352]
                    tunnel: w328 -> [_ w351]
                    tunnel: w336 -> [w348 w350]
                    tunnel: [w348 w349] -> w335
                    frame False {
                    }
                    frame True {
                      n241 = Increment(x=w352) -> (x+1=w355:i32)
                      n242 = Divide(x=w352, y=w355) -> (x/y=w353:dbl)
                      n243 = Divide(x=w351, y=w355) -> (x/y=w356:dbl[])
                      n244 = Multiply(x=w350, y=w353) -> (x*y=w354:dbl[])
                      n245 = Add(x=w354, y=w356) -> (x+y=w349:dbl[])
                      n246 = local write "Average of Scans"(w349) -> ()
                    }
                  }
                }
                n247 = Concatenate Strings("}" ("string"), "\r\n") -> (w297:string)
                n248 = Write to Text File(file (use dialog)=w300, text=w297) -> (refnum out=w301:refnum<file>)  [unwired: 2 in, 2 out]
                n249 = Close File(refnum=w301) -> ()  [unwired: 1 in, 2 out]
              }
            }
          }
          event "Fit": Value Change {
            n250 = event-data() -> ("NewVal"=w417:bool)  [unwired: 1 in, 4 out]
            n251 = case shown="True" w417 {
              frame False {
              }
              frame True {
                n252 = local write "Fit"(FALSE ("Fit")) -> ()
                n253 = property on="Average Counts or States" class="WFChart (strict)"() -> ("History Data"=→"History Data":dbl[])  [unwired: 2 in, 2 out]
              }
            }
          }
          event "Clear": Value Change {
            n254 = event-data() -> ()  [unwired: 1 in, 6 out]
            n255 = property on="Average Counts or States" class="WFChart (strict)"("History Data"=dbl[] []) -> ()  [unwired: 2 in, 2 out]
          }
          event "Sequence File": Value Change {
            n256 = event-data() -> ("NewVal"=w422:path)  [unwired: 1 in, 4 out]
            n257 = call <vilib>:"Check if File or Folder Exists.vi"("path"=w422) -> ("file or folder exists?"=w423:bool, "dup path"=w421:path)  [unwired: 8 in, 1 out]
            n258 = case shown="True" w423 {
              tunnel: w421 -> [_ w424]
              frame False {
              }
              frame True {
                n259 = flat-sequence {
                  tunnel: w424 -> [w428]
                  frame #0 {
                    n260 = Read from Text File(file (use dialog)=w428) -> (text=w429:string)  [unwired: 3 in, 3 out]
                    n261 = call "LoadSequenceString.vi"("Sequence String"=w429) -> ("Chapter"=w427:string, "Sequence"=w426:string)
                    n262 = local write "Chapter (us)"(w427) -> ()
                    n263 = call "CompileSequence.vi"("Sequence"=w426, "Chapter"=w427) -> ("Compiled Sequence"=w425:string)
                    n264 = local write "Sequence"(w426) -> ()
                    n265 = local write "CompiledSequence"(w425) -> ()
                  }
                  frame #1 {
                    n266 = property on="Compile" class="Bool (strict)"("Val(Sgnl)"=TRUE ("Value (Signaling)")) -> ()  [unwired: 2 in, 2 out]
                  }
                }
              }
            }
          }
          event "Sweep": Value Change {
            n267 = event-data() -> ("NewVal"=w435:bool)  [unwired: 1 in, 4 out]
            n268 = case shown="True" w435 {
              tunnel: w434 -> [_ w440]
              tunnel: w433 -> [_ _]
              tunnel: w432 -> [_ w439]
              tunnel: w431 -> [_ w438]
              frame False {
              }
              frame True {
                n269 = flat-sequence {
                  tunnel: w440 -> [w450]
                  tunnel: w439 -> [w445]
                  tunnel: w438 -> [w444]
                  tunnel: [w443] -> w437
                  tunnel: ["Save"] -> w436
                  tunnel: w437 -> [w467]
                  tunnel: w436 -> [w465]
                  frame #0 {
                    w451 = dbl[] [] ("History Data")
                    w448 = 0.0 ("X Scale.Offset and Multiplier:Offset")
                    w449 = 1.0 ("X Scale.Offset and Multiplier:Multiplier")
                    n270 = property on="Average Counts or States" class="WFChart (strict)"("History Data"=w451, "Height"=w450) -> (error out=w446:errorcluster)  [unwired: 2 in, 1 out]
                    n271 = property on="Average of Scans" class="WFGraph (strict)"("XScale.Multiplier"=w449, "XScale.Offset"=w448, "XScale.Maximum"=0.0 ("X Scale.Range:Maximum"), "Value"=w451) -> ()  [unwired: 2 in, 2 out]
                    n272 = case shown="True" "Save" {
                      tunnel: ["" w462] -> w442
                      tunnel: w445 -> [_ w459]
                      tunnel: w444 -> [_ w456]
                      tunnel: [_ w455] -> w443
                      frame False {
                      }
                      frame True {
                        n273 = local read "Chapter (us)"() -> (w461:string)
                        n274 = local read "Sequence"() -> (w457:string)
                        n275 = call "NewData.vi"("Prefix"="Sweep-") -> ("data file name"=w462:string, "data file refnum"=w460:refnum<file>)  [unwired: 2 in]
                        n276 = call "SaveSequenceString.vi"("Sequence"=w457, "Chapter"=w461) -> ("Sequence String"=w458:string)
                        n277 = Format Into String(format string=w459, initial string=w460, w458) -> (resulting string=w454:refnum<file>)  [unwired: 1 in, 1 out]
                        n278 = Write to Text File(file (use dialog)=w454, text=w456) -> (refnum out=w455:refnum<file>)  [unwired: 2 in, 2 out]
                      }
                    }
                    n279 = property on="Average Counts or States" class="WFChart (strict)"(error in=w446, "XScale.Multiplier"=w449, "XScale.Offset"=w448, "XScale.Maximum"=100.0 ("X Scale.Range:Maximum")) -> ()  [unwired: 1 in, 2 out]
                    n280 = local write "data file"(w442) -> ()
                  }
                  frame #1 {
                    n281 = while {
                      tunnel: [w474] -> w466
                      tunnel: w467 -> [w473]
                      tunnel: w465 -> [w472]
                      tunnel: [w472] -> w464
                      i -> [w471]
                      stop <- w475 continue-if-true
                      n282 = flat-sequence {
                        tunnel: [w481] -> w474
                        tunnel: w473 -> [w480]
                        tunnel: w472 -> [w479]
                        tunnel: w471 -> [w478]
                        frame #0 {
                          n283 = property on="Data" class="Bool (strict)"("Val(Sgnl)"=TRUE ("Value (Signaling)")) -> ()  [unwired: 2 in, 2 out]
                        }
                        frame #1 {
                          n284 = while {
                            stop <- w477 continue-if-true
                            n285 = local read "Data"() -> (w477:bool)
                          }
                        }
                        frame #2 {
                          n286 = case shown="True" w479 {
                            tunnel: [w482 w487] -> w481
                            tunnel: w480 -> [w482 w486]
                            tunnel: w478 -> [_ w483]
                            frame False {
                            }
                            frame True {
                              n287 = local read "Counts"() -> (w491:u32[])
                              n288 = Format Into String(format string="%d One,", w483) -> (resulting string=w484:string)  [unwired: 2 in, 1 out]
                              n289 = for {
                                tunnel: w491 -> [w496] mode=indexing
                                shift-right: [w494] -> w490
                                shift-left: w484 -> [w493]
                                n290 = Number To Decimal String(number=w496) -> (decimal integer string=w495:string)  [unwired: 1 in]
                                n291 = call <vilib>:"Space Constant.vi"() -> ("String"=w492:string)
                                n292 = Concatenate Strings(w493, w492, w495) -> (w494:string)
                              }
                              n293 = Concatenate Strings(w490, "\r\n") -> (w488:string)
                              n294 = Write to Text File(file (use dialog)=w486, text=w488) -> (refnum out=w487:refnum<file>)  [unwired: 2 in, 2 out]
                            }
                          }
                        }
                      }
                      n295 = local read "Sweep"() -> (w475:bool)
                    }
                    n296 = case shown="True" w464 {
                      tunnel: w466 -> [_ w469]
                      frame False {
                      }
                      frame True {
                        n297 = Write to Text File(file (use dialog)=w469, text="}\n") -> (refnum out=w470:refnum<file>)  [unwired: 2 in, 2 out]
                        n298 = Close File(refnum=w470) -> ()  [unwired: 1 in, 2 out]
                      }
                    }
                  }
                }
              }
            }
          }
          event "Sequencer": Value Change {
            n299 = event-data() -> ("NewVal"=w497:bool)  [unwired: 1 in, 4 out]
          }
        }
      }
    }
    frame #2 {
      n300 = local read "Sequencer Port"() -> (w498:refnum<visa-resource-name>)
      n301 = VISA Close(VISA resource name=w498) -> ()  [unwired: 1 in, 1 out]
    }
  }
